vi "TemperatureVaporTank.vi"(11 "Temp. Voltage\n[V]":dbl) -> (3 "Temp. []":dbl)   [LabVIEW 2017]
uses:
  <vilib>/express/express arith-compare/Formula/XNode/ExpressFormulaBlockNode.xnode
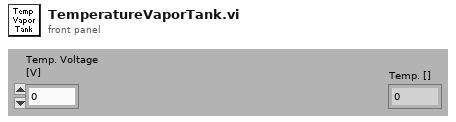
[diagram p1: front panel]
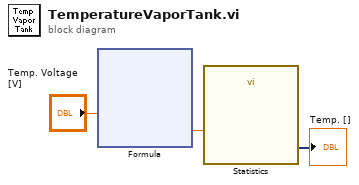
[diagram p0: block diagram]
diagram:
  n1 = xnode "Formula"("V"="Temp. Voltage\n[V]") -> ("Result"=w2:dbl)  [unwired: 1 in, 1 out]
  n2 = call "Statistics"("Signals"=w2) -> ("Arithmetic Mean"=→"Temp. []":dynamicdata)  [unwired: 25 in, 1 out]
